vi "ME45_HW1.vi"() -> ()   [LabVIEW 2023]
uses:
  <vilib>/Analysis/5stat.llb/RMS (DBL).vi
  <vilib>/express/express analysis/Spectral/Block/exnSpectralBlock spectral measurements RMS poly.vi
  <vilib>/express/express analysis/Spectral/Block/exnSpectralBlock spectral measurements RMS DDT.vi
  <vilib>/express/express analysis/Spectral/XNode/ExpressSpectralMeasurementsBlockNode.xnode
  <vilib>/Analysis/NI_AALPro.lvlib
panel:
  in  "stop 2":bool
  out "Ring":u16(ring)
  out "Sound Pressure (dB)":dbl(knob) scale=0.0..100.0
  in  "Sample Rate (Hz)":dbl(slide) scale=11025.0..96000.0
  in  "stop":bool
  in  "FFT":dynamicdata(graph)=[{"t0"=timestamp(0 s since 1904-01-01), "dt"=1.0000084803256446, "Y"=array[22000 elements], "attributes"=variant("NI_ChannelName"=variant(string "Filtered (FFT - (RMS))"), "NI_OriginalChannelName"=variant(string "Filtered"))}]
  in  "Microphone Input":dynamicdata(graph)=[{"t0"=timestamp(3789231291.814481 s since 1904-01-01), "dt"=2.2727079994233427e-05, "Y"=array[44000 elements]}]
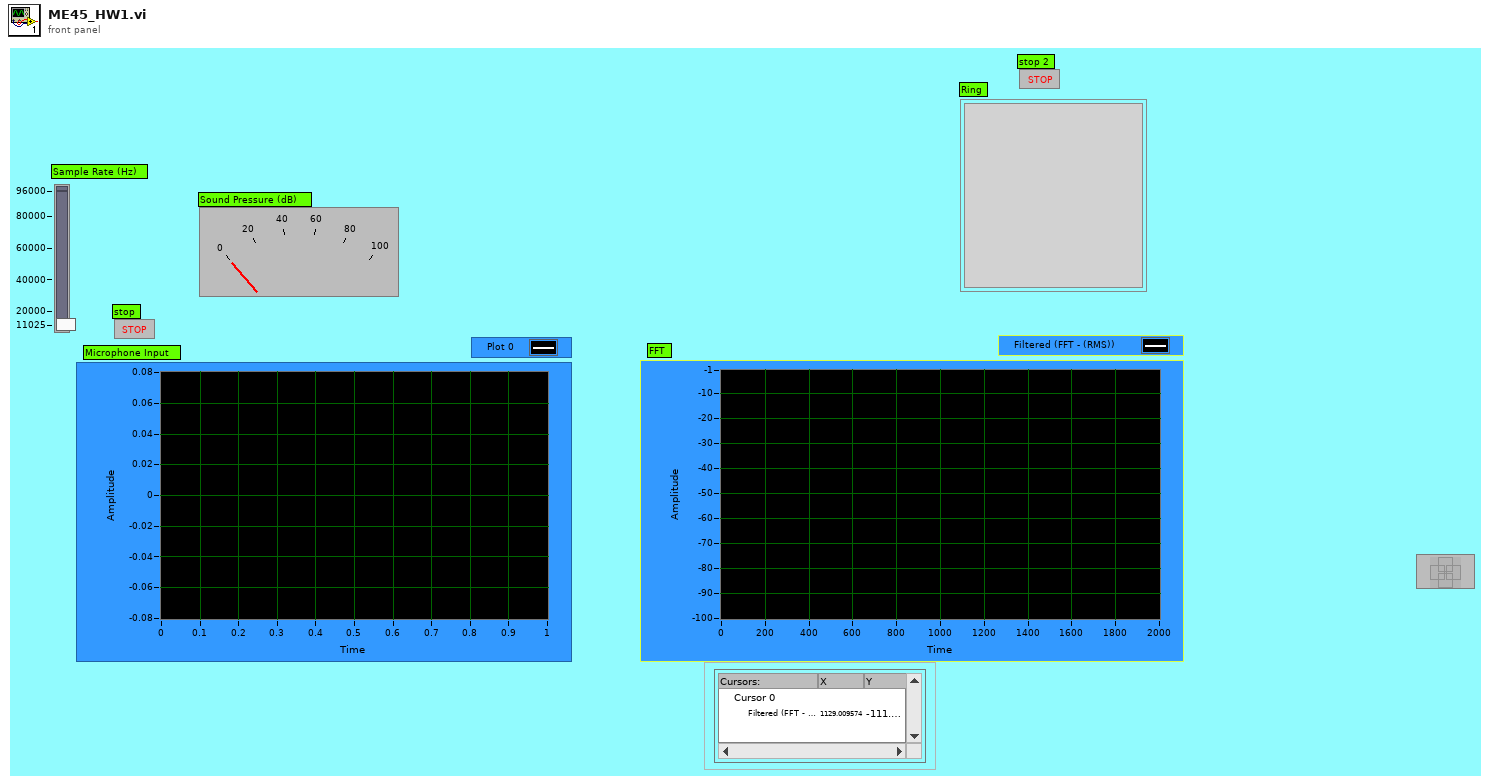
[diagram p1: front panel]
types:
  T1 = cluster{"averaging mode":u16, "weighting mode":u16, "number of averages":u32}
  T2 = cluster{"dB On (F)":bool, "unwrap phase (F)":bool, "convert to degree (F)":bool}
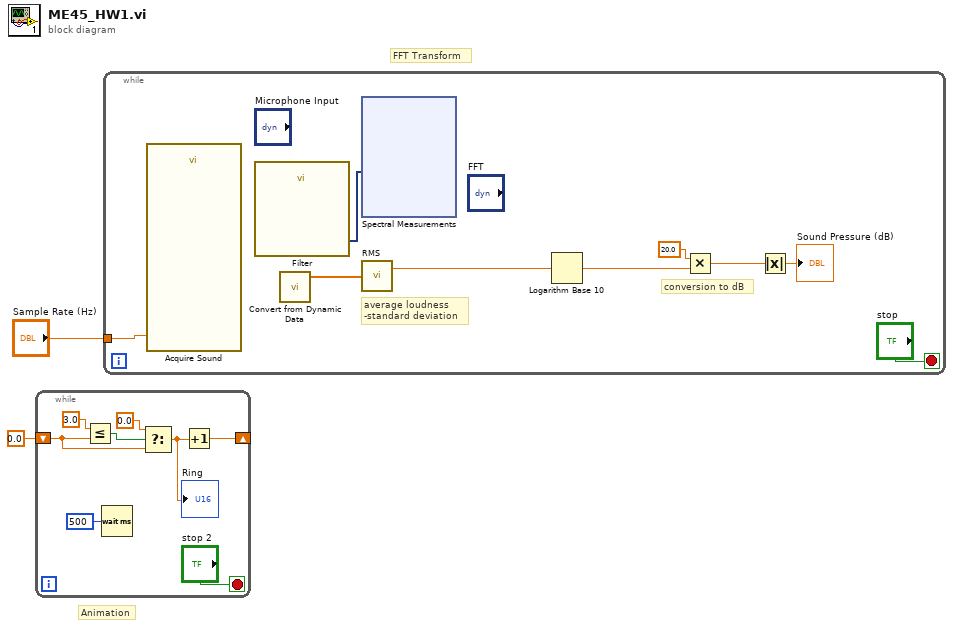
[diagram p0: block diagram]
diagram:
  # "FFT Transform"
  # "Animation"
  n1 = while {
    shift-right: [w8] -> _
    shift-left: 0.0 -> [w7]
    stop <- "stop 2" stop-if-true
    n2 = Less Or Equal?(x=3.0, y=w7) -> (x <= y?=w9:bool)
    n3 = Wait (ms)(milliseconds to wait=u32 500) -> ()  [unwired: 1 out]
    n4 = Select(t=0.0, s=w9, f=w7) -> (s? t:f=w4:dbl)
    "Ring" <- w4
    n5 = Increment(x=w4) -> (x+1=w8:dbl)
  }
  n6 = while {
    tunnel: "Sample Rate (Hz)" -> [w18]
    stop <- "stop" stop-if-true
    # "conversion to dB"
    # "average loudness \n-standard deviation"
    n7 = call "Acquire Sound"("Sample rate (Hz)"=w18) -> ()  [unwired: 17 in, 2 out]
    n8 = call "Filter"() -> ("Filtered Signal"=w19:dynamicdata)  [unwired: 10 in, 1 out]
    n9 = call "Convert from Dynamic Data"() -> ("Array"=w16:dbl[])  [unwired: 4 in]
    n10 = xnode "Spectral Measurements"("Signals"=w19) -> ()  [unwired: 1 in, 3 out]
    n11 = call-poly <vilib>:"RMS.vi"("X"=w16) -> ("rms value"=w14:dbl)  [unwired: 1 out]
    n12 = Logarithm Base 10(1:w14) -> (0:w13:dbl)
    n13 = Multiply(x=20.0, y=w13) -> (x*y=w12:dbl)
    n14 = Absolute Value(x=w12) -> (abs(x)=→"Sound Pressure (dB)":dbl)
  }
